vi "Write configuration.vi"(8 "error in (no error)":errorcluster, 10 "configuration":refnum<class "CEF_serializable configuration.lvclass">, 11 "Abstract Engine in":refnum<class "Abstract Engine.lvclass">) -> (0 "error out":errorcluster, 3 "Abstract Engine out":refnum<class "Abstract Engine.lvclass">)   [LabVIEW 2025, in "Abstract Engine.lvlib" / "Abstract Engine.lvclass"]
uses:
  Abstract Engine.lvclass
  Users/Public/Documents/Sandia National Labs/TSS Plugin/CEF.lvlibp/serializable configuration/CEF_serializable configuration.lvclass
  Engine configuration/Engine configuration.lvclass
  Abstract Engine.lvclass/Abstract Engine.ctl
panel:
  # "!st child should be overrided, which inherited from serial node"
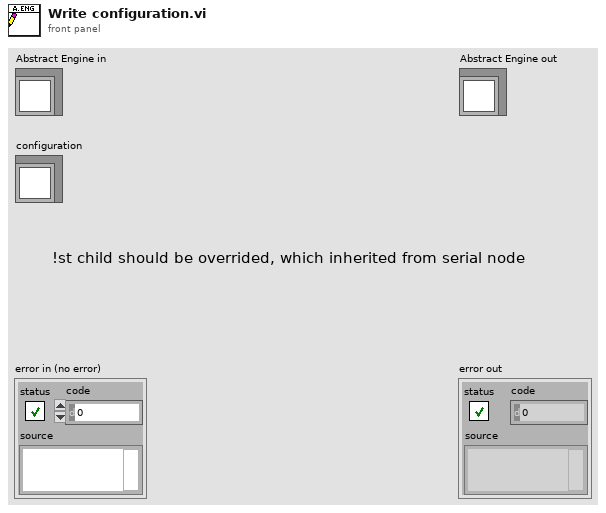
[diagram p1: front panel]
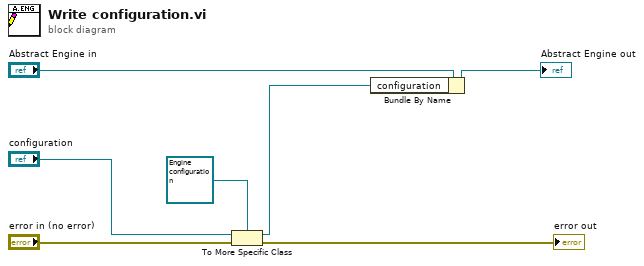
[diagram p0: block diagram]
diagram:
  n1 = To More Specific Class(target class=refnum<class "Engine configuration.lvclass"> refnum ("Engine configuration.lvclass"), reference="configuration", error in="error in (no error)") -> (specific class reference=w1:refnum<class "Engine configuration.lvclass">, error out=→"error out":errorcluster)
  n2 = Bundle By Name(cluster="Abstract Engine in", "configuration"=w1) -> (→"Abstract Engine out":refnum<class "Abstract Engine.lvclass">)
